vi "Update Test Info.vi"(8 "error in (no error)":errorcluster, 11 "Test Information":T1={"APU Part Number:"="555", "Model:"="5", "Serial Number:"="sad", "Customer:"="sad", "Work Order:"="asd", "Pre or Post SB"="Pre SB 49-7711", "Run Count"=0, "APU Selected"="<Select>"} {"Run Count" min=0 step=1}) -> (0 "error out":errorcluster)   [LabVIEW 2018, in "Testing UI 1.lvlib"]
doc: "This subVI enqueues the named action in to the communications queue along with the input data."
uses:
  Testing UI 1.lvlib
  Controller (Host)/Public Controls/Test Information.ctl
  Controller (Host)/Public VIs/PreorPostSB.ctl
  Controller (Host)/Public Controls/APU Select.ctl
  Private Controls/Module Action.ctl
  Private Controls/Module Data.ctl
  Controller (Host)/Controller (Host).lvlib
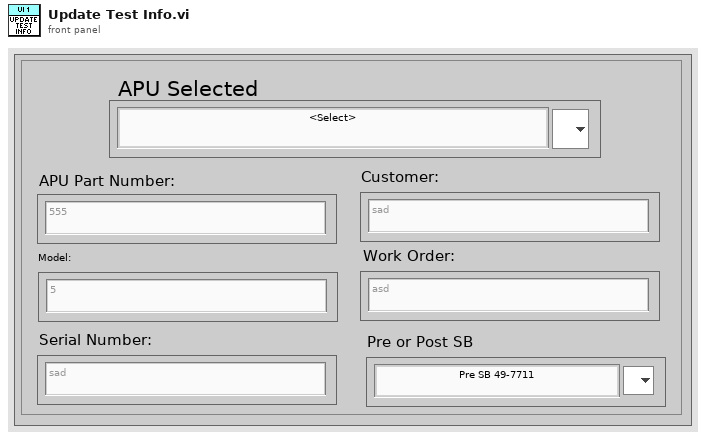
[diagram p1: front panel]
types:
  T1 = typedef "Controller (Host).lvlib/Test Information.ctl" = cluster{"APU Part Number:":string, "Model:":string, "Serial Number:":string, "Customer:":string, "Work Order:":string, "Pre or Post SB":T2, "Run Count":i32, "APU Selected":T3}
  T2 = typedef "Controller (Host).lvlib/PreorPostSB.ctl" = string
  T3 = typedef "Controller (Host).lvlib/APU Select.ctl" = string
  T4 = typedef "Testing UI 1.lvlib/Module Action.ctl" = enum8{"Init", "Open FP", "Timeout", "New Report Value", "Update Test Info", "Record Data", "Update Report Path", "SetFuelPressure", "Error", "Exit", "Update System Log", "Load APU Setup Data", "Threshold ALERT", "Engine Start Val Change", "Value to Record"}
  T5 = typedef "Testing UI 1.lvlib/Module Data.ctl" = cluster{"Data":variant, "Action":T4}
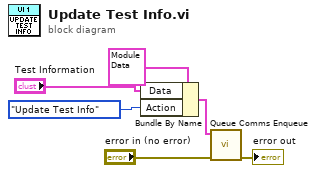
[diagram p0: block diagram]
diagram:
  n1 = Bundle By Name(cluster=T5 {"Data"=variant, "Action"=enum."Init"} ("element"), "Data"="Test Information", "Action"=Module_Action."Update Test Info") -> (w6:T5)
  n2 = call "Queue Comms Enqueue.vi"("error in (no error)"="error in (no error)", "element"=w6) -> ("error out"=→"error out":errorcluster)  [unwired: 9 in]
